vi "initialaize.vi"(8 "error in (no error)":errorcluster, 9 "Visa com port":refnum<visa-resource-name>, 10 "Serial Device Brand":T1, 11 "Cypress in":refnum<class "Cypress.lvclass">) -> (0 "error out":errorcluster, 3 "Cypress out":refnum<class "Cypress.lvclass">)   [LabVIEW 2020, in "Cypress.lvclass"]
uses:
  Cypress.lvclass
  Combo box/serial device brand.ctl
  <vilib>/Instr/_visa.llb/VISA Configure Serial Port (Instr).vi
  Abstracts/Serial Device/Serial Device.lvclass
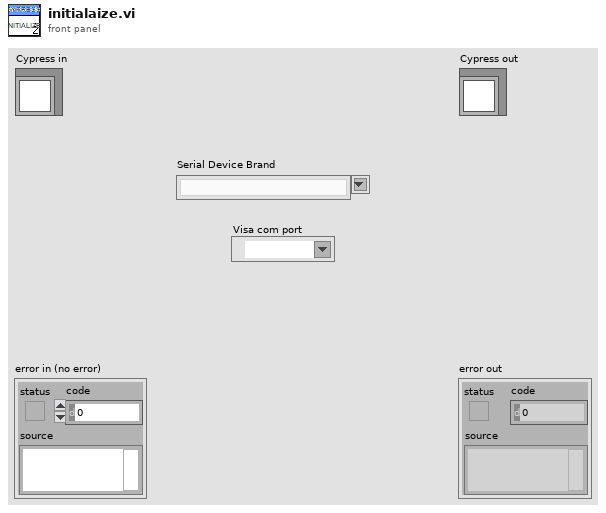
[diagram p1: front panel]
types:
  T1 = typedef "Serial Device.lvclass/serial device brand.ctl" = string
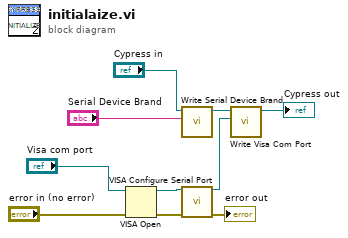
[diagram p0: block diagram]
diagram:
  n1 = VISA Open(error in (no error)="error in (no error)", VISA resource name="Visa com port") -> (VISA resource name=w7:refnum<visa-resource-name>, error out=w9:errorcluster)  [unwired: 3 in]
  n2 = call-dynamic "Write Serial Device Brand.vi"("Serial Device Brand"="Serial Device Brand", "Serial Device in"="Cypress in") -> ("Serial Device out"=w5:refnum<class "Cypress.lvclass">)  [unwired: 8 in, 1 out]
  n3 = call-poly "VISA Configure Serial Port"("VISA resource name"=w7, "error in (no error)"=w9) -> ("VISA resource name out"=w1:refnum<visa-resource-name>, "error out"=→"error out":errorcluster)  [unwired: 12 in]
  n4 = call-dynamic "Write Visa Com Port.vi"("Visa Com Port"=w1, "Serial Device in"=w5) -> ("Serial Device out"=→"Cypress out":refnum<class "Cypress.lvclass">)  [unwired: 8 in, 1 out]
